vi "SetParam.vi"(8 "error in (no error)":errorcluster caption="entrée d'erreur (pas d'erreur)", 10 "MaxAbsScaler":cluster{"copy":bool}={"copy"=TRUE}, 11 "MaxAbsScaler.lvclass":refnum<class "MaxAbsScaler.lvclass">) -> (0 "error out":errorcluster caption="sortie d'erreur", 3 "MaxAbsScaler.lvclass":refnum<class "MaxAbsScaler.lvclass">)   [LabVIEW 2020, in "MaxAbsScaler.lvclass"]
doc: "Set Parameters"
uses:
  MaxAbsScaler.lvclass
  MaxAbsScaler.lvclass/MaxAbsScaler.ctl
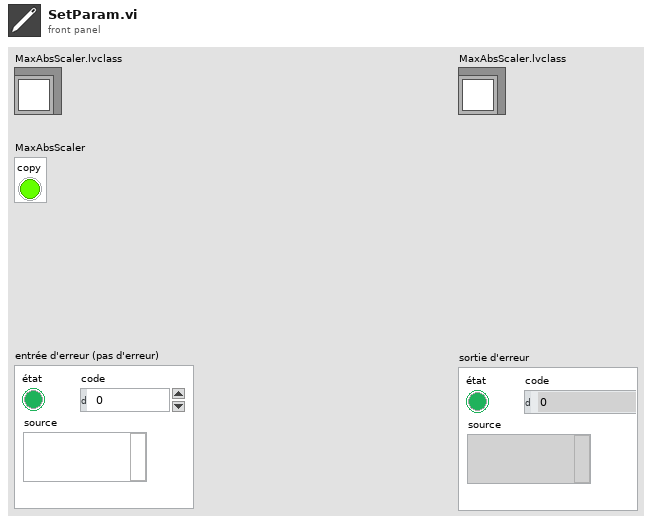
[diagram p1: front panel]
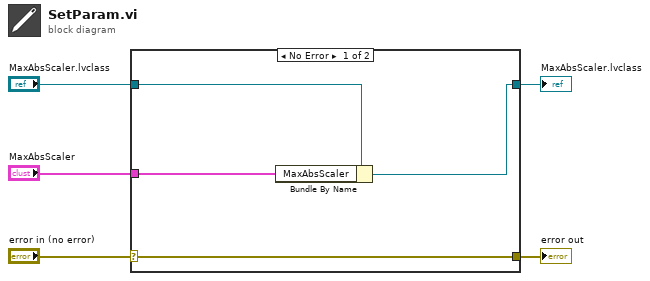
[diagram p0: block diagram]
diagram:
  n1 = case shown="No Error" "error in (no error)" {
    selector: "error in (no error)" -> [w9 w10]
    tunnel: [w9 w10] -> w4
    tunnel: [w7 w11] -> w2
    tunnel: "MaxAbsScaler.lvclass" -> [w8 w11]
    tunnel: "MaxAbsScaler" -> [w6 _]
    frame No Error {
      n2 = Bundle By Name(cluster=w8, "MaxAbsScaler"=w6) -> (w7:refnum<class "MaxAbsScaler.lvclass">)
    }
    frame Error {
    }
  }
  "error out" <- w4
  "MaxAbsScaler.lvclass" <- w2
